vi "daqmx_linear_current.vi"() -> ()   [LabVIEW 2019]
uses:
  <vilib>/DAQmx/create/channels.llb/DAQmx Create Channel (AI-Current-Basic).vi
  <vilib>/DAQmx/configure/timing.llb/DAQmx Timing (Sample Clock).vi
  <vilib>/DAQmx/configure/task.llb/DAQmx Configure Logging (TDMS).vi
panel:
  out "data":waveform(dbl)={"t0"=timestamp(3653046944.881683 s since 1904-01-01), "dt"=0.001, "Y"=[1.3113022632182994e-08, 1.3113022632182994e-08, 1.3113022632182994e-08, 1.3113022632182994e-08, 1.3113022632182994e-08, 1.3113022632182994e-08, 1.3113022632182994e-08, 1.3113022632182994e-08, 1.3113022632182994e-08, 1.3113022632182994e-08], "attributes"=variant("NI_ChannelName"=variant(string "NI9208/ai0"), "NI_UnitDescription"=variant(string "Amps"))}
  in  "NI-9208":tag="NI9208/ai0"
  out "Error Out":errorcluster
  in  "TDMS File":path=path "C:/Python/projects/nitdms/tests/tdms_files/daqmx_linear_current.tdms"
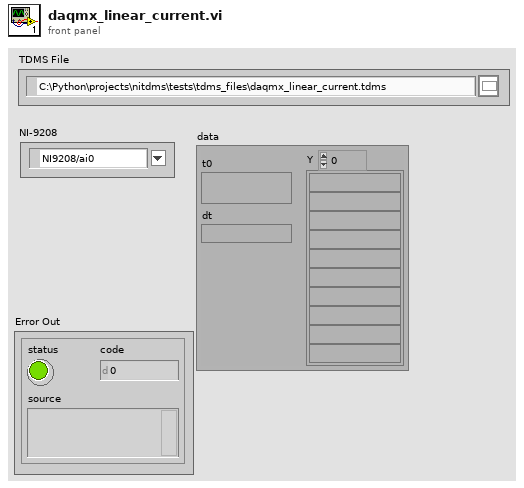
[diagram p1: front panel]
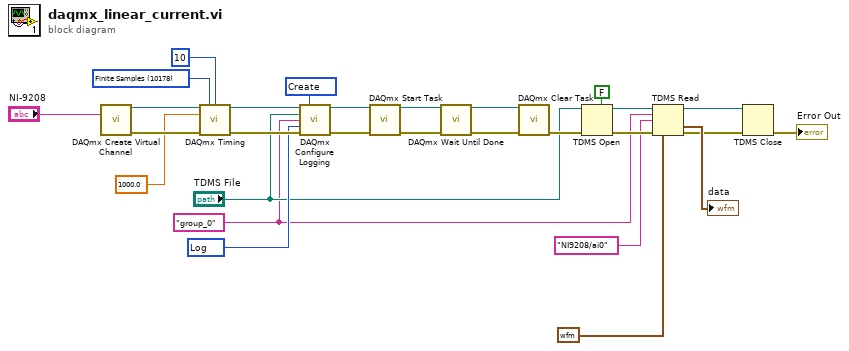
[diagram p0: block diagram]
diagram:
  w19 = 10178 items=["Finite Samples"=10178, "Continuous Samples"=10123, "Hardware Timed Single Point"=12522] ("sample mode")
  w22 = 15844 items=["Off"=10231, "Log"=15844, "Log and Read"=15842] ("logging mode")
  w8 = "group_0" ("group name")
  w23 = 15848 items=["Open"=10437, "Open or Create"=15846, "Create or Replace"=15847, "Create"=15848] ("operation")
  n1 = call-poly <vilib>:"DAQmx Create Virtual Channel.vi"("physical channels"="NI-9208") -> ("task out"=w27:refnum<k21>, "error out"=w28:errorcluster)  [unwired: 13 in]
  n2 = call-poly <vilib>:"DAQmx Timing.vi"("task/channels in"=w27, "sample mode"=w19, "samples per channel"=10, "rate"=1000.0, "error in"=w28) -> ("task out"=w24:refnum<k21>, "error out"=w25:errorcluster)  [unwired: 9 in]
  n3 = call-poly <vilib>:"DAQmx Configure Logging.vi"("task/channels in"=w24, "operation"=w23, "file path"="TDMS File", "group name"=w8, "logging mode"=w22, "error in"=w25) -> ("task out"=w20:refnum<k21>, "error out"=w21:errorcluster)  [unwired: 8 in]
  n4 = call <vilib>:"DAQmx Start Task.vi"("task/channels in"=w20, "error in"=w21) -> ("task out"=w16:refnum<k21>, "error out"=w17:errorcluster)  [unwired: 12 in]
  n5 = call <vilib>:"DAQmx Wait Until Done.vi"("task/channels in"=w16, "error in"=w17) -> ("task out"=w14:refnum<k21>, "error out"=w15:errorcluster)  [unwired: 12 in]
  n6 = call <vilib>:"DAQmx Clear Task.vi"("task in"=w14, "error in"=w15) -> ("error out"=w13:errorcluster)  [unwired: 13 in]
  n7 = TDMS Open(5:FALSE ("create index file? (T)"), 8:w13, 11:"TDMS File") -> (0:w10:errorcluster, 3:w9:refnum<k34>)  [unwired: 4 in]
  n8 = TDMS Read(0:w9, 5:w8, 7:"NI9208/ai0" ("channel name(s) in"), 11:w10, 12:waveform(dbl) {"t0"=timestamp(0 s since 1904-01-01), "dt"=1.0, "Y"=[]} ("Waveform")) -> (4:w2:refnum<k34>, 10:→"data":waveform(dbl), 15:w3:errorcluster)  [unwired: 3 in, 3 out]
  n9 = TDMS Close(8:w3, 11:w2) -> (0:→"Error Out":errorcluster)  [unwired: 1 out]
